vi "Write DI Scope Data.vi"(8 "error in (no error)":errorcluster, 10 "DI Scope Data":sgl[][](array[numeric]), 11 "DCM-DSI-HW in":refnum<class "DCM-DSI.lvclass">) -> (0 "error out":errorcluster, 3 "DCM-DSI-HW out":refnum<class "DCM-DSI.lvclass">)   [LabVIEW 2016, in "DCM-DSI.lvclass"]
uses:
  DCM-DSI.lvclass
  DCM-DSI.lvclass/DCM-DSI.ctl
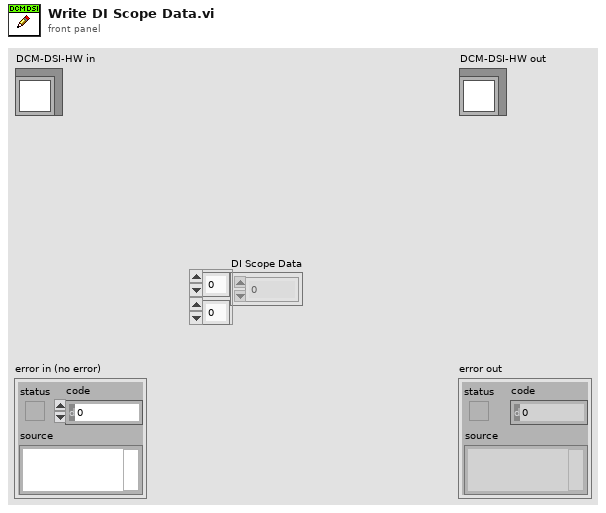
[diagram p1: front panel]
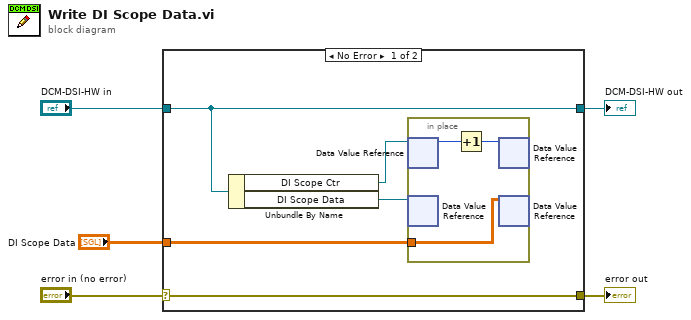
[diagram p0: block diagram]
diagram:
  n1 = case shown="No Error" "error in (no error)" {
    selector: "error in (no error)" -> [w10 w15]
    tunnel: [w10 w15] -> w4
    tunnel: [w8 w14] -> w2
    tunnel: "DCM-DSI-HW in" -> [w8 w14]
    tunnel: "DI Scope Data" -> [w7 _]
    frame No Error {
      n2 = Unbundle By Name(w8) -> ("DI Scope Ctr"=w6:refnum<data-value>, "DI Scope Data"=w9:refnum<data-value>)
      n3 = in-place {
        in-place-border: w7 -> [w13]
        n4 = in-place-dvr #1(w6) -> (w12:u32)  [unwired: 1 out]
        n5 = in-place-dvr #2(w9) -> ()  [unwired: 2 out]
        n6 = Increment(x=w12) -> (x+1=w11:u32)
        n7 = in-place-dvr #1(w11) -> ()  [unwired: 2 out]
        n8 = in-place-dvr #2(w13) -> ()  [unwired: 2 out]
      }
    }
    frame Error {
    }
  }
  "error out" <- w4
  "DCM-DSI-HW out" <- w2
